vi "MPU_Stick_Get_Write_Parameters.vi"() -> ()   [LabVIEW 2017]
uses:
  <vilib>/Utility/file.llb/Read Delimited Spreadsheet (string).vi
panel:
  out "C header file defines":string
  out "Write parameters":string[](array[string])
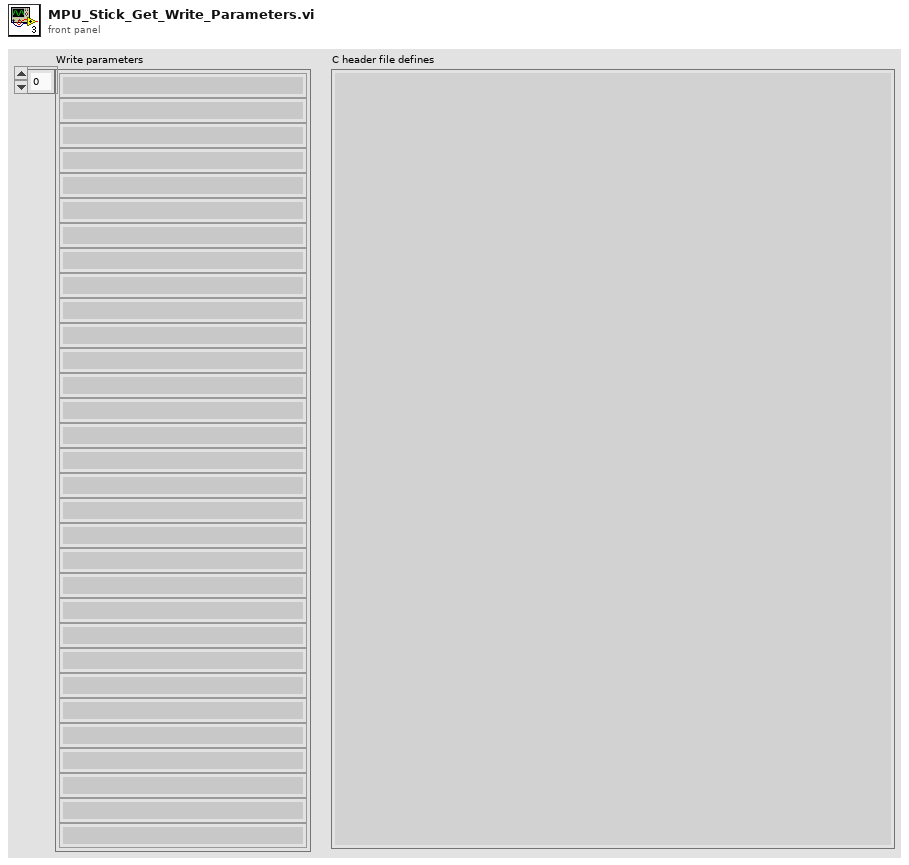
[diagram p1: front panel]
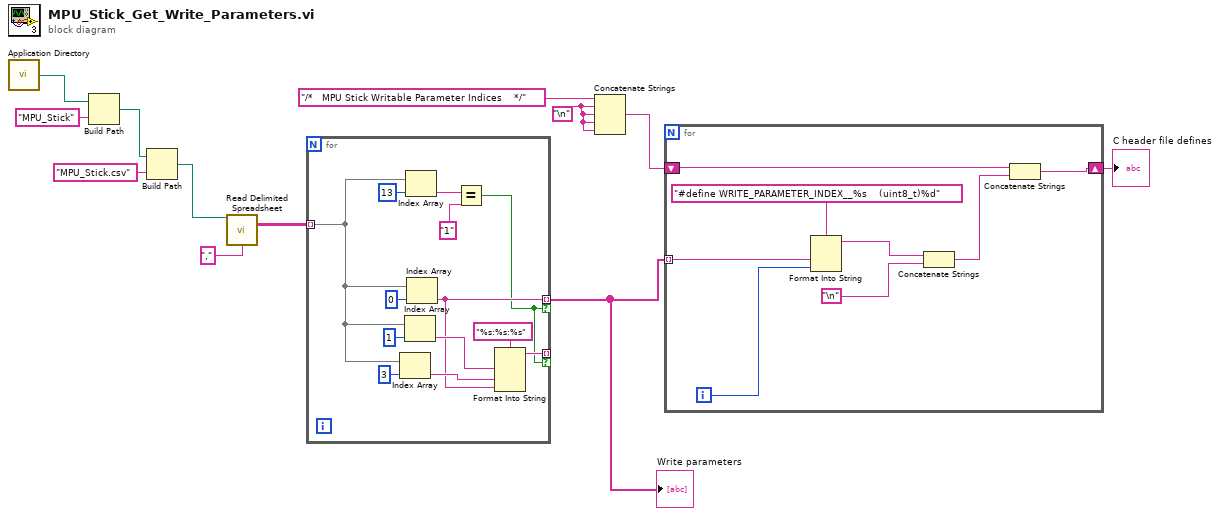
[diagram p0: block diagram]
diagram:
  w3 = "\n"
  n1 = call <vilib>:"Application Directory.vi"() -> ("Application Directory"=w12:path)
  n2 = Build Path(base path=w12, name or relative path="MPU_Stick") -> (appended path=w10:path)
  n3 = Build Path(base path=w10, name or relative path="MPU_Stick.csv") -> (appended path=w8:path)
  n4 = call-poly <vilib>:"Read Delimited Spreadsheet.vi"("file path (dialog if empty)"=w8, "delimiter (\\t)"="," ("delimiter (\\t)")) -> ("all rows"=w6:string[][])  [unwired: 8 in, 5 out]
  n5 = for {
    tunnel: w6 -> [w19] mode=indexing
    tunnel: [w15] -> w1 mode=indexing if=w13
    tunnel: [w14] -> _ mode=indexing if=w13
    n6 = Index Array(array=w19, index=3) -> (element=w16:string)
    n7 = Index Array(array=w19, index=1) -> (element=w17:string)
    n8 = Index Array(array=w19, index=13) -> (element=w24:string)
    n9 = Index Array(array=w19, index=0) -> (element=w15:string)
    n10 = Equal?(x=w24, y="1") -> (x = y?=w13:bool)
    n11 = Format Into String(format string="%s:%s:%s", w17, w16, w15) -> (resulting string=w14:string)  [unwired: 2 in, 1 out]
  }
  "Write parameters" <- w1
  n12 = Concatenate Strings("/*   MPU Stick Writable Parameter Indices    */", w3, w3, w3, w3) -> (w2:string)
  n13 = for {
    shift-right: [w27] -> w5
    shift-left: w2 -> [w29]
    tunnel: w1 -> [w26] mode=indexing
    i -> [w32]
    n14 = Format Into String(format string="#define WRITE_PARAMETER_INDEX__%s    (uint8_t)%d", w26, w32) -> (resulting string=w31:string)  [unwired: 2 in, 1 out]
    n15 = Concatenate Strings(w31, "\n") -> (w28:string)
    n16 = Concatenate Strings(w29, w28) -> (w27:string)
  }
  "C header file defines" <- w5
